vi "Write to TDMS Log File (Waveform).vi"(6 "Waveform Data":waveform(dbl)[](array[waveform]), 8 "error in (no error)":errorcluster, 9 "Channel Names in":string[](array[string]), 10 "Group Names in":string[](array[string]), 11 "TDMS Log File in":refnum<class "TDMS Log File.lvclass">) -> (0 "error out":errorcluster, 3 "TDMS Log File out":refnum<class "TDMS Log File.lvclass">)   [LabVIEW 2015, in "TDMS Log File.lvclass"]
uses:
  TDMS Log File.lvclass
  TDMS Log File.lvclass/TDMS Log File.ctl
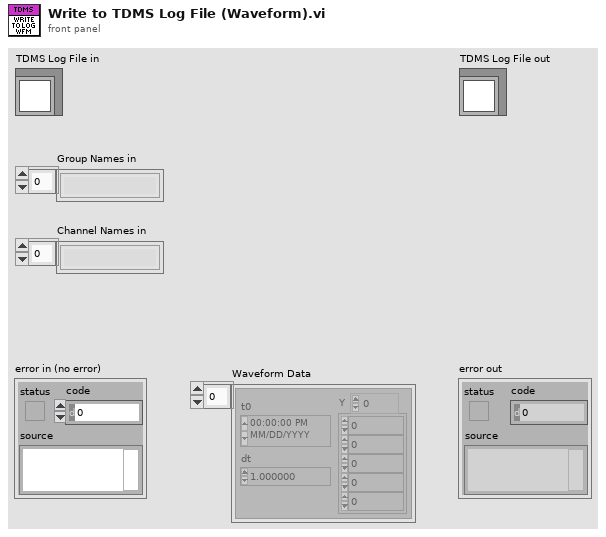
[diagram p1: front panel]
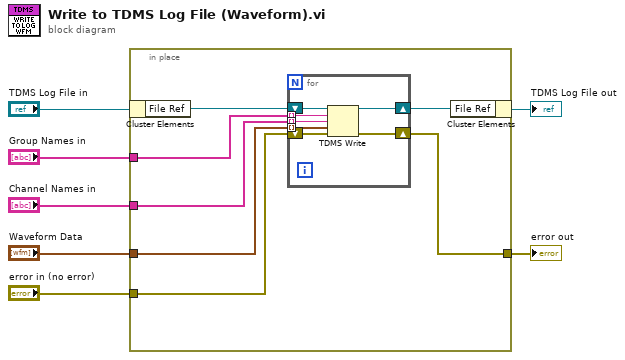
[diagram p0: block diagram]
diagram:
  n1 = in-place {
    in-place-border: "Group Names in" -> [w13]
    in-place-border: "Channel Names in" -> [w12]
    in-place-border: "Waveform Data" -> [w11]
    in-place-border: "error in (no error)" -> [w9]
    in-place-border: [w8] -> w1
    n2 = in-place-cluster #1("TDMS Log File in") -> ("File Ref"=w14:refnum<k34>)
    n3 = for {
      tunnel: w13 -> [w20] mode=indexing
      tunnel: w12 -> [w19] mode=indexing
      tunnel: w11 -> [w18] mode=indexing
      shift-right: [w17] -> w10
      shift-left: w14 -> [w21]
      shift-right: [w15] -> w8
      shift-left: w9 -> [w16]
      n4 = TDMS Write(0:w21, 5:w20, 7:w19, 9:w18, 11:w16) -> (4:w17:refnum<k34>, 15:w15:errorcluster)  [unwired: 1 in, 2 out]
    }
    n5 = in-place-cluster #1("File Ref"=w10) -> (→"TDMS Log File out":refnum<class "TDMS Log File.lvclass">)
  }
  "error out" <- w1
